vi "Main.vi"() -> ()   [LabVIEW 2017]
doc: "The myRIO Project template acquires acceleration data from the onboard accelerometer and displays the changes of acceleration values in a waveform chart."
uses:
  <vilib>/myRIO/Common/Instrument Driver Framework/myRIO v1.0/Encoder/typedefs/Encoder Count Direction Enum.ctl
  Motor Status Enum.ctl
  <vilib>/myRIO/Instrument Drivers/Onboard IO/PWM/typedefs/PWM Reference.ctl
  <vilib>/myRIO/Common/Instrument Driver Framework/Utilities/typedefs/myRIO Generic Hardware Reference.ctl
  <vilib>/myRIO/Common/Instrument Driver Framework/Utilities/typedefs/Hardware Version Enum.ctl
  <vilib>/myRIO/Common/Instrument Driver Framework/Utilities/typedefs/myRIO v1.0 Reference.ctl
  <vilib>/myRIO/Common/Instrument Driver Framework/Utilities/typedefs/Generic FPGA Reference.ctl
  <vilib>/myRIO/Common/Instrument Driver Framework/myRIO v1.0/PWM/typedefs/PWM Channels Enum.ctl
  <vilib>/myRIO/Instrument Drivers/Onboard IO/PWM/typedefs/PWM Configuration.ctl
  <vilib>/userdefined/High Color/nirio_resource_hc.ctl
  <vilib>/myRIO/Common/Instrument Driver Framework/Utilities/vis/Is FPGA Ref Available.vi
  <vilib>/myRIO/Common/Instrument Driver Framework/myRIO v1.0/PWM/vis/myRIO v1.1 Open PWM.vi
  <vilib>/myRIO/Instrument Drivers/Onboard IO/PWM/vis/Set Duty Cycle and Frequency.vi
  <vilib>/myRIO/Common/Instrument Driver Framework/Utilities/vis/Validate Channels.vi
  <vilib>/myRIO/Common/Instrument Driver Framework/myRIO v1.0/PWM/vis/myRIO v1.0 Reserve PWM.vi
  <vilib>/myRIO/Common/Instrument Driver Framework/myRIO v1.0/UART/vis/myRIO v1.0 Close UART.vi
  <vilib>/myRIO/Common/Instrument Driver Framework/myRIO v1.0/PWM/vis/myRIO v1.0 Build MUX Configuration PWM.vi
  <vilib>/myRIO/Common/Instrument Driver Framework/myRIO v1.0/Resource Manager/vis/myRIO v1.0 Reserve Channel List.vi
  <vilib>/myRIO/Common/Instrument Driver Framework/myRIO v1.0/Resource Manager/vis/myRIO v1.0 Create Configuration List.vi
  <vilib>/myRIO/Common/Instrument Driver Framework/myRIO v1.0/Resource Manager/vis/myRIO v1.0 Reserve Channel.vi
  <vilib>/myRIO/Common/Instrument Driver Framework/myRIO v1.0/Resource Manager/vis/myRIO v1.0 Unreserve Channel.vi
  <vilib>/myRIO/Common/Instrument Driver Framework/myRIO v1.0/Resource Manager/vis/myRIO v1.0 Build Mutex Name.vi
  <vilib>/Utility/VariantDataType/GetNumericInfo.vi
  <vilib>/Utility/error.llb/Error Cluster From Error Code.vi
  <vilib>/myRIO/Common/Instrument Driver Framework/myRIO v1.0/myRIO v1.1 Open.vi
  <vilib>/myRIO/Common/Instrument Driver Framework/Utilities/vis/IO Manager.vi
  <vilib>/myRIO/Common/Instrument Driver Framework/Utilities/vis/Configuration Manager.vi
  <vilib>/myRIO/Common/Instrument Driver Framework/myRIO v1.0/Resource Manager/vis/myRIO v1.0 Configure IO.vi
  <vilib>/myRIO/Common/Instrument Driver Framework/myRIO v1.0/myRIO v1.0 Close.vi
  <vilib>/myRIO/Common/Instrument Driver Framework/myRIO v1.0/PWM/vis/myRIO v1.0 Write PWM.vi
  <vilib>/myRIO/Common/Instrument Driver Framework/Utilities/vis/FPGA Ref Manager.vi
  <vilib>/myRIO/Common/Instrument Driver Framework/myRIO v1.0/myRIO v1.0 Reset FPGA.vi
  <vilib>/myRIO/Common/Instrument Driver Framework/myRIO v1.0/IRQ/vis/myRIO v1.0 IRQ Info FGV.vi
  <vilib>/myRIO/Common/Instrument Driver Framework/myRIO v1.0/IRQ/vis/myRIO v1.0 Timer IRQ Info FGV.vi
  <vilib>/myRIO/Common/Instrument Driver Framework/myRIO v1.0/IRQ/vis/myRIO v1.0 ISR Agent.vi
  <vilib>/myRIO/Express VI/Onboard IO/PWM/PWM Express VI.xnode
  <vilib>/myRIO/Instrument Drivers/Onboard IO/PWM/vis/myRIO PWM Open.xnode
  <vilib>/myRIO/Instrument Drivers/Utilities/Utilities.lvlib
  <vilib>/myRIO/Instrument Drivers/Onboard IO/PWM/PWM.lvlib
panel:
  out "X Axis state":T1
  out "Y Axis state":T1
  out "Loop Runtime (s)":dbl format="%.3f"
  in  "Clear Chart History":bool
  in  "Coordinates Input":cluster{"X-axis (mm)":dbl, "Y-axis (mm)":dbl}
  out "Y Axis":T2(graph)
  out "X Axis":T2(graph)
  in  "X Axis Motor Target":T3
  out "X Axis Motor Params":T4
  in  "Y Axis Motor Target":T5
  out "Y Axis Motor Params":T5
  in  "stop":bool
  out "Output String":string
  out "Encoder Output":T7
  out "Total Runtime (s)":dbl format="%.2f"
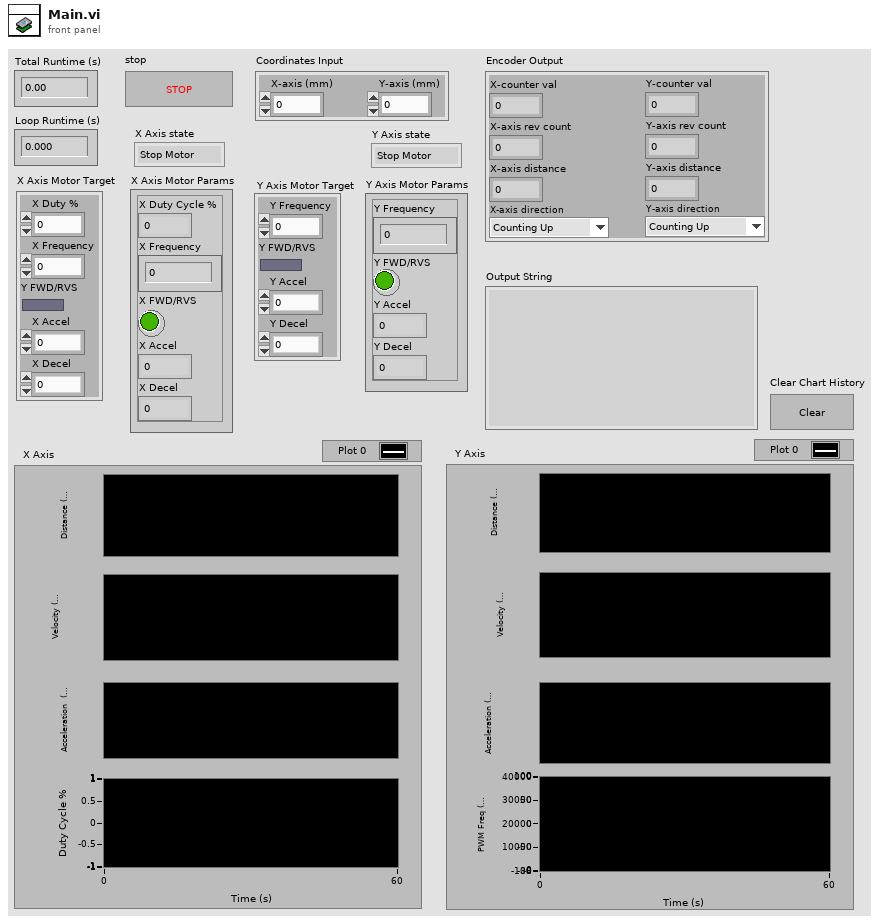
[diagram p1: front panel]
types:
  T1 = typedef "Motor Status Enum.ctl" = enum16{"Stop Motor", "Read Inputs", "Steady Speed", "Accelerate", "Decelerate"}
  T2 = cluster{"X-axis distance":dbl, dbl, dbl, "X Frequency":dbl}
  T3 = cluster{"X Frequency":dbl, "Y FWD/RVS":bool, "X Accel":dbl, "X Decel":dbl, "X Duty %":dbl}
  T4 = cluster{"X Frequency":dbl, "X FWD/RVS":bool, "X Accel":dbl, "X Decel":dbl, "X Duty Cycle %":dbl}
  T5 = cluster{"Y Frequency":dbl, "Y FWD/RVS":bool, "Y Accel":dbl, "Y Decel":dbl}
  T6 = typedef "Encoder Count Direction Enum.ctl" = enum16{"Counting Up", "Counting Down"}
  T7 = cluster{"Y-axis rev count":dbl, "Y-axis distance":dbl, "X-axis rev count":dbl, "X-axis distance":dbl, "Y-axis direction":T6, "X-axis direction":T6, "X-counter val":i32, "Y-counter val":i32}
  T8 = cluster{"X-axis distance":dbl, dbl, dbl, "X Frequency":dbl}[]
  T9 = cluster{dbl, dbl, "X-axis distance":dbl, "X Duty Cycle %":dbl, "X Frequency":dbl, "Y-axis distance":dbl, "Y Frequency":dbl, "X Accel":dbl, "X Decel":dbl, "Y Accel":dbl, "Y Decel":dbl, "X-axis (mm)":dbl, "Y-axis (mm)":dbl, dbl, dbl, dbl, dbl}
  T10 = cluster{"X-axis distance":dbl, dbl, dbl, "X Duty Cycle %":dbl}
  T11 = cluster{"Y-axis distance":dbl, dbl, dbl, "Y Frequency":dbl}
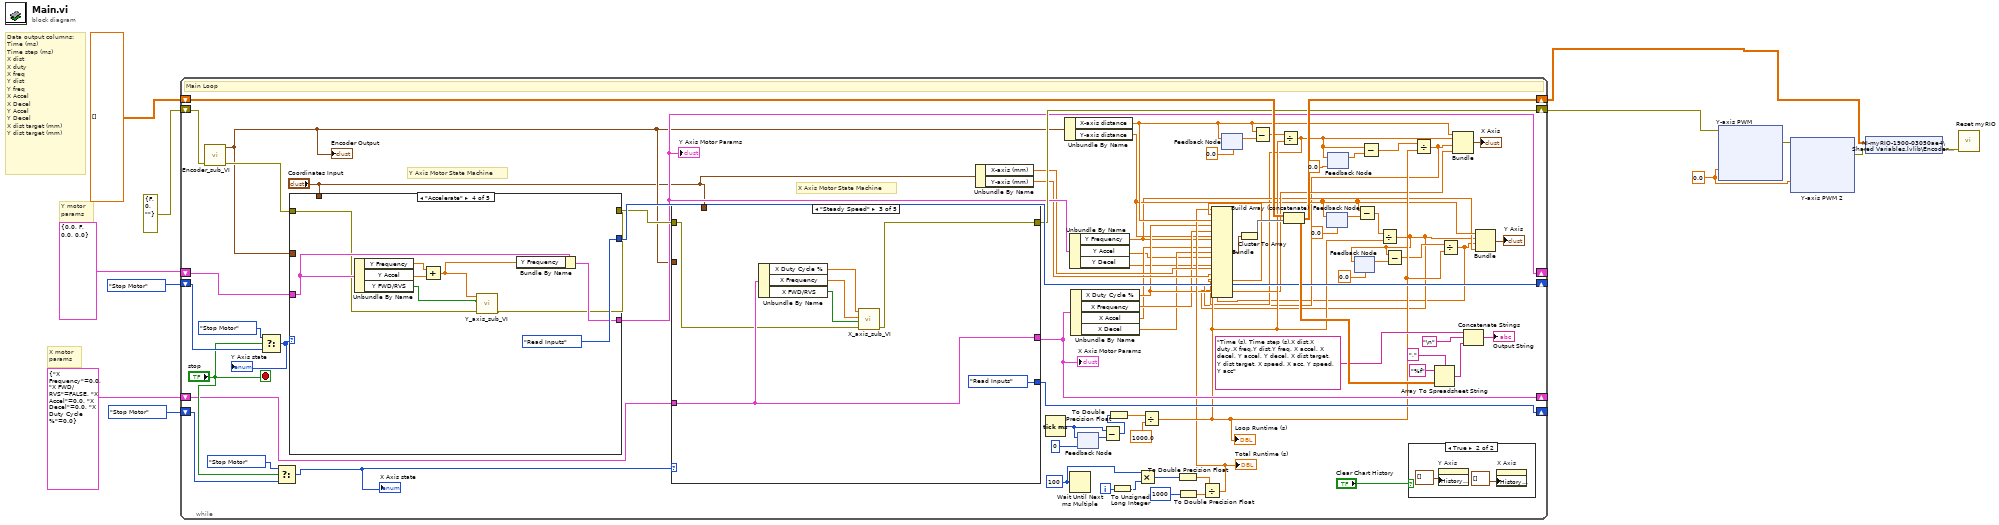
[diagram p0: block diagram]
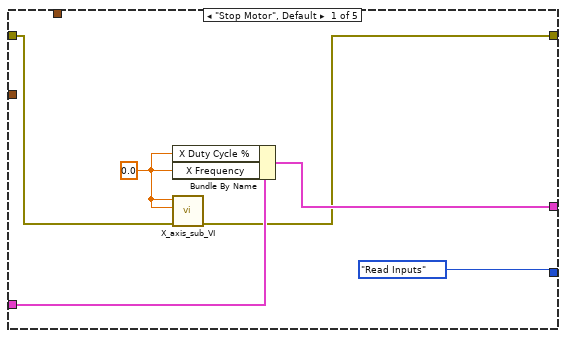
[diagram p3: hidden frame]
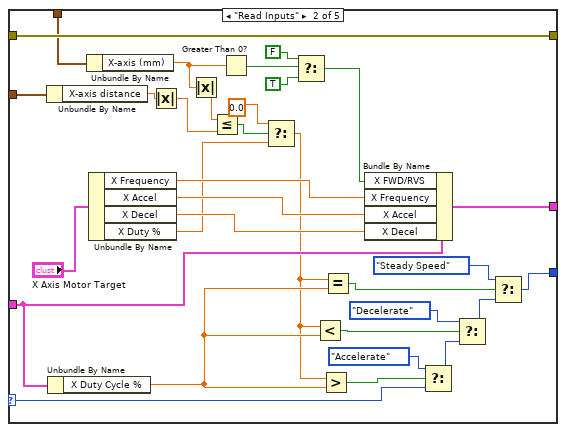
[diagram p4: hidden frame]
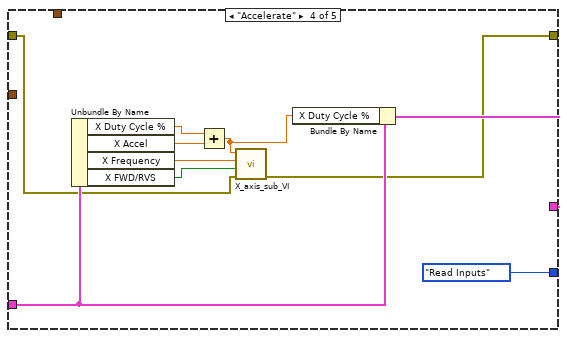
[diagram p5: hidden frame]
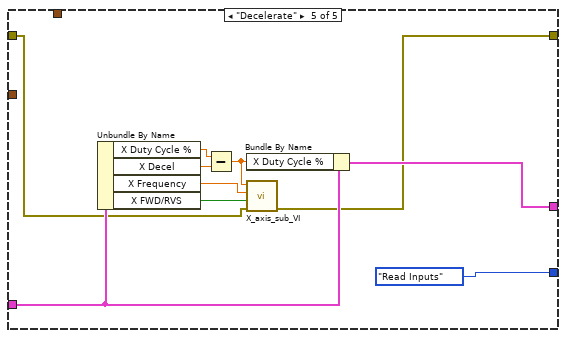
[diagram p6: hidden frame]
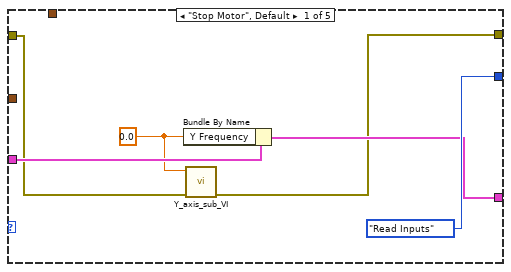
[diagram p7: hidden frame]
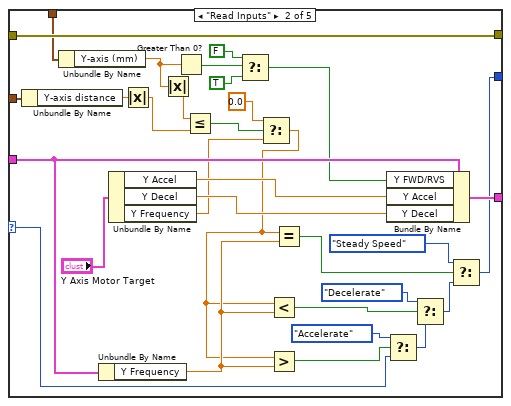
[diagram p8: hidden frame]
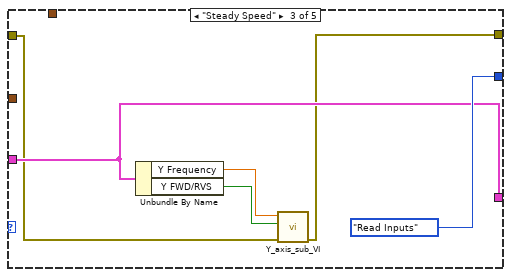
[diagram p9: hidden frame]
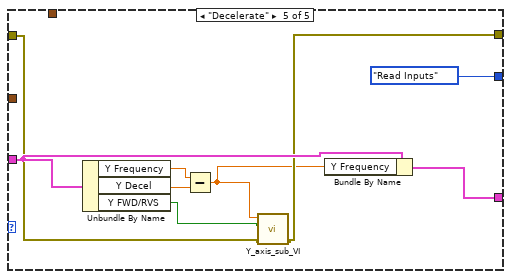
[diagram p10: hidden frame]
diagram:
  w6 = 0.0 ("Frequency [Hz]")
  # "X motor \nparams"
  # "Y motor \nparams"
  # "Data output columns:\nTime (ms)\nTime step (ms)\nX dist\nX duty\nX freq\nY dist\nY freq\nX Accel\nX Decel\nY Accel\nY Decel\nX dist target (mm)\nY dist target (mm)"
  n1 = while {
    shift-right: [w68] -> w12
    shift-left: errorcluster {"status"=FALSE, "code"=0, "source"=""} ("error in (no error)") -> [w86]
    shift-right: [w83] -> w1
    shift-left: dbl[][] [] -> [w82]
    shift-right: [w60] -> _
    shift-left: T5 {"Y Frequency"=0.0, "Y FWD/RVS"=FALSE, "Y Accel"=0.0, "Y Decel"=0.0} ("Y Axis Motor Params 2") -> [w81]
    shift-right: [w80] -> _
    shift-left: Motor_Status_Enum."Stop Motor" -> [w78]
    shift-right: [w71] -> _
    shift-left: Motor_Status_Enum."Stop Motor" -> [w73]
    shift-right: [w61] -> _
    shift-left: T4 {"X Frequency"=0.0, "X FWD/RVS"=FALSE, "X Accel"=0.0, "X Decel"=0.0, "X Duty Cycle %"=0.0} ("X Axis Motor Params 3") -> [w70]
    i -> [w32]
    stop <- "stop" stop-if-true
    w31 = u32 100 ("milliseconds to wait")
    # "X Axis Motor State Machine"
    # "Y Axis Motor State Machine"
    # "Main Loop"
    n2 = call "Encoder_sub_VI.vi"("error in (no error)"=w86) -> ("error out"=w76:errorcluster, "Encoder Output"=w59:T7)  [unwired: 9 in]
    "Encoder Output" <- w59
    n3 = Select(t=Motor_Status_Enum."Stop Motor", s="stop", f=w78) -> (s? t:f=w79:T1)
    "Y Axis state" <- w79
    n4 = Select(t=Motor_Status_Enum."Stop Motor", s="stop", f=w73) -> (s? t:f=w74:T1)
    "X Axis state" <- w74
    n5 = case shown="\"Accelerate\"" w79 {
      selector: w79 -> [_ w176 _ _ _]
      tunnel: w81 -> [w159 w177 w193 w202 w210]
      tunnel: [Motor_Status_Enum."Read Inputs" w160 Motor_Status_Enum."Read Inputs" Motor_Status_Enum."Read Inputs" Motor_Status_Enum."Read Inputs"] -> w80
      tunnel: [w157 w178 w193 w201 w211] -> w60
      tunnel: w76 -> [w155 w175 w192 w198 w208]
      tunnel: [w156 w175 w191 w197 w209] -> w69
      tunnel: w59 -> [_ w174 _ _ _]
      tunnel: "Coordinates Input" -> [_ w170 _ _ _]
      frame "Stop Motor", Default {
        w154 = 0.0 ("Y Frequency")
        n6 = Bundle By Name(cluster=w159, "Y Frequency"=w154) -> (w157:T5)
        n7 = call "Y_axis_sub_VI.vi"("error in (no error)"=w155, "Frequency"=w154) -> ("error out"=w156:errorcluster)  [unwired: 9 in]
      }
      frame "Read Inputs" {
        n8 = Unbundle By Name(w174) -> ("Y-axis distance"=w168:dbl)
        n9 = Unbundle By Name(w170) -> ("Y-axis (mm)"=w167:dbl)
        n10 = Unbundle By Name(w177) -> ("Y Frequency"=w184:dbl)
        n11 = Unbundle By Name("Y Axis Motor Target") -> ("Y Accel"=w188:dbl, "Y Decel"=w189:dbl, "Y Frequency"=w162:dbl)
        n12 = Absolute Value(x=w168) -> (abs(x)=w165:dbl)
        n13 = Absolute Value(x=w167) -> (abs(x)=w166:dbl)
        n14 = Greater Than 0?(x=w167) -> (x > 0?=w169:bool)
        n15 = Less Or Equal?(x=w166, y=w165) -> (x <= y?=w164:bool)
        n16 = Select(t=FALSE, s=w169, f=TRUE) -> (s? t:f=w171:bool)
        n17 = Select(t=0.0, s=w164, f=w162) -> (s? t:f=w161:dbl)
        n18 = Less?(x=w161, y=w184) -> (x < y?=w181:bool)
        n19 = Greater?(x=w161, y=w184) -> (0:w190:bool)
        n20 = Equal?(x=w161, y=w184) -> (x = y?=w185:bool)
        n21 = Bundle By Name(cluster=w177, "Y FWD/RVS"=w171, "Y Accel"=w188, "Y Decel"=w189) -> (w178:T5)
        n22 = Select(t=Motor_Status_Enum."Accelerate", s=w190, f=w176) -> (s? t:f=w183:T1)
        n23 = Select(t=Motor_Status_Enum."Decelerate", s=w181, f=w183) -> (s? t:f=w186:T1)
        n24 = Select(t=Motor_Status_Enum."Steady Speed", s=w185, f=w186) -> (s? t:f=w160:T1)
      }
      frame "Steady Speed" {
        n25 = Unbundle By Name(w193) -> ("Y Frequency"=w195:dbl, "Y FWD/RVS"=w196:bool)
        n26 = call "Y_axis_sub_VI.vi"("error in (no error)"=w192, "FWD/RVS"=w196, "Frequency"=w195) -> ("error out"=w191:errorcluster)  [unwired: 8 in]
      }
      frame "Accelerate" {
        n27 = Unbundle By Name(w202) -> ("Y Frequency"=w204:dbl, "Y Accel"=w205:dbl, "Y FWD/RVS"=w199:bool)
        n28 = Add(x=w204, y=w205) -> (x+y=w200:dbl)
        n29 = call "Y_axis_sub_VI.vi"("error in (no error)"=w198, "FWD/RVS"=w199, "Frequency"=w200) -> ("error out"=w197:errorcluster)  [unwired: 8 in]
        n30 = Bundle By Name(cluster=w202, "Y Frequency"=w200) -> (w201:T5)
      }
      frame "Decelerate" {
        n31 = Unbundle By Name(w210) -> ("Y Frequency"=w214:dbl, "Y Decel"=w213:dbl, "Y FWD/RVS"=w207:bool)
        n32 = Subtract(x=w214, y=w213) -> (x-y=w206:dbl)
        n33 = call "Y_axis_sub_VI.vi"("error in (no error)"=w208, "FWD/RVS"=w207, "Frequency"=w206) -> ("error out"=w209:errorcluster)  [unwired: 8 in]
        n34 = Bundle By Name(cluster=w210, "Y Frequency"=w206) -> (w211:T5)
      }
    }
    "Y Axis Motor Params" <- w60
    n35 = case shown="\"Steady Speed\"" w74 {
      selector: w74 -> [_ w114 _ _ _]
      tunnel: [Motor_Status_Enum."Read Inputs" w107 Motor_Status_Enum."Read Inputs" Motor_Status_Enum."Read Inputs" Motor_Status_Enum."Read Inputs"] -> w71
      tunnel: [w91 w113 w130 w137 w147] -> w61
      tunnel: w70 -> [w92 w112 w130 w136 w146]
      tunnel: w69 -> [w90 w110 w128 w135 w145]
      tunnel: [w89 w110 w127 w134 w144] -> w68
      tunnel: w59 -> [_ w109 _ _ _]
      tunnel: "Coordinates Input" -> [_ w108 _ _ _]
      frame "Stop Motor", Default {
        w94 = 0.0 ("Y Frequency")
        n36 = Bundle By Name(cluster=w92, "X Duty Cycle %"=w94, "X Frequency"=w94) -> (w91:T4)
        n37 = call "X_axis_sub_VI.vi"("error in (no error)"=w90, "Frequency"=w94, "Duty Cycle %"=w94) -> ("error out"=w89:errorcluster)  [unwired: 8 in]
      }
      frame "Read Inputs" {
        n38 = Unbundle By Name(w109) -> ("X-axis distance"=w101:dbl)
        n39 = Unbundle By Name(w112) -> ("X Duty Cycle %"=w125:dbl)
        n40 = Unbundle By Name(w108) -> ("X-axis (mm)"=w99:dbl)
        n41 = Unbundle By Name("X Axis Motor Target") -> ("X Frequency"=w117:dbl, "X Accel"=w115:dbl, "X Decel"=w116:dbl, "X Duty %"=w97:dbl)
        n42 = Absolute Value(x=w101) -> (abs(x)=w100:dbl)
        n43 = Absolute Value(x=w99) -> (abs(x)=w104:dbl)
        n44 = Less Or Equal?(x=w104, y=w100) -> (x <= y?=w103:bool)
        n45 = Greater Than 0?(x=w99) -> (x > 0?=w105:bool)
        n46 = Select(t=0.0, s=w103, f=w97) -> (s? t:f=w96:dbl)
        n47 = Select(t=FALSE, s=w105, f=TRUE) -> (s? t:f=w98:bool)
        n48 = Less?(x=w96, y=w125) -> (x < y?=w120:bool)
        n49 = Greater?(x=w96, y=w125) -> (0:w118:bool)
        n50 = Equal?(x=w96, y=w125) -> (x = y?=w124:bool)
        n51 = Bundle By Name(cluster=w112, "X FWD/RVS"=w98, "X Frequency"=w117, "X Accel"=w115, "X Decel"=w116) -> (w113:T4)
        n52 = Select(t=Motor_Status_Enum."Accelerate", s=w118, f=w114) -> (s? t:f=w122:T1)
        n53 = Select(t=Motor_Status_Enum."Decelerate", s=w120, f=w122) -> (s? t:f=w123:T1)
        n54 = Select(t=Motor_Status_Enum."Steady Speed", s=w124, f=w123) -> (s? t:f=w107:T1)
      }
      frame "Steady Speed" {
        n55 = Unbundle By Name(w130) -> ("X Duty Cycle %"=w132:dbl, "X Frequency"=w131:dbl, "X FWD/RVS"=w133:bool)
        n56 = call "X_axis_sub_VI.vi"("error in (no error)"=w128, "FWD/RVS"=w133, "Frequency"=w131, "Duty Cycle %"=w132) -> ("error out"=w127:errorcluster)  [unwired: 7 in]
      }
      frame "Accelerate" {
        n57 = Unbundle By Name(w136) -> ("X Duty Cycle %"=w139:dbl, "X Accel"=w140:dbl, "X Frequency"=w141:dbl, "X FWD/RVS"=w143:bool)
        n58 = Add(x=w139, y=w140) -> (x+y=w142:dbl)
        n59 = call "X_axis_sub_VI.vi"("error in (no error)"=w135, "FWD/RVS"=w143, "Frequency"=w141, "Duty Cycle %"=w142) -> ("error out"=w134:errorcluster)  [unwired: 7 in]
        n60 = Bundle By Name(cluster=w136, "X Duty Cycle %"=w142) -> (w137:T4)
      }
      frame "Decelerate" {
        n61 = Unbundle By Name(w146) -> ("X Duty Cycle %"=w149:dbl, "X Decel"=w150:dbl, "X Frequency"=w151:dbl, "X FWD/RVS"=w153:bool)
        n62 = Subtract(x=w149, y=w150) -> (x-y=w152:dbl)
        n63 = Bundle By Name(cluster=w146, "X Duty Cycle %"=w152) -> (w147:T4)
        n64 = call "X_axis_sub_VI.vi"("error in (no error)"=w145, "FWD/RVS"=w153, "Frequency"=w151, "Duty Cycle %"=w152) -> ("error out"=w144:errorcluster)  [unwired: 7 in]
      }
    }
    "X Axis Motor Params" <- w61
    n65 = Unbundle By Name("Coordinates Input") -> ("X-axis (mm)"=w25:dbl, "Y-axis (mm)"=w50:dbl)
    n66 = Tick Count (ms)() -> (millisecond timer value=w49:u32)
    n67 = Unbundle By Name(w59) -> ("X-axis distance"=w46:dbl, "Y-axis distance"=w20:dbl)
    n68 = Unbundle By Name(w60) -> ("Y Frequency"=w19:dbl, "Y Accel"=w18:dbl, "Y Decel"=w17:dbl)
    n69 = Wait Until Next ms Multiple(millisecond multiple=w31) -> ()  [unwired: 1 out]
    n70 = Unbundle By Name(w61) -> ("X Duty Cycle %"=w24:dbl, "X Frequency"=w23:dbl, "X Accel"=w22:dbl, "X Decel"=w21:dbl)
    n71 = feedback-in #1(w49) -> ()
    n72 = feedback #1(u32 0) -> (w48:u32)
    n73 = Subtract(x=w49, y=w48) -> (x-y=w54:u32)
    n74 = To Double Precision Float(number=w54) -> (double precision float=w52:dbl)
    n75 = To Unsigned Long Integer(number=w32) -> (unsigned 32bit integer=w30:u32)
    n76 = Multiply(x=w31, y=w30) -> (x*y=w29:u32)
    n77 = Divide(x=w52, y=1000.0) -> (x/y=w37:dbl)
    "Loop Runtime (s)" <- w37
    n78 = To Double Precision Float(number=w29) -> (double precision float=w27:dbl)
    n79 = To Double Precision Float(number=u32 1000 ("y")) -> (double precision float=w26:dbl)
    n80 = Divide(x=w27, y=w26) -> (x/y=w28:dbl)
    "Total Runtime (s)" <- w28
    n81 = feedback #2(0.0) -> (w45:dbl)
    n82 = feedback-in #2(w46) -> ()
    n83 = Subtract(x=w46, y=w45) -> (x-y=w44:dbl)
    n84 = Divide(x=w44, y=w37) -> (x/y=w16:dbl)
    n85 = feedback #3(0.0) -> (w40:dbl)
    n86 = feedback-in #3(w20) -> ()
    n87 = feedback #4(0.0) -> (w43:dbl)
    n88 = feedback-in #4(w16) -> ()
    n89 = feedback #5(0.0) -> (w35:dbl)
    n90 = Subtract(x=w20, y=w40) -> (x-y=w38:dbl)
    n91 = Subtract(x=w16, y=w43) -> (x-y=w41:dbl)
    n92 = Divide(x=w38, y=w37) -> (x/y=w14:dbl)
    n93 = feedback-in #5(w14) -> ()
    n94 = Subtract(x=w14, y=w35) -> (x-y=w34:dbl)
    n95 = case shown="True" "Clear Chart History" {
      frame False {
      }
      frame True {
        n96 = property on="Y Axis" class="WFChart (strict)"("History Data"=T8 []) -> ()  [unwired: 2 in, 2 out]
        n97 = property on="X Axis" class="WFChart (strict)"("History Data"=T8 []) -> ()  [unwired: 2 in, 2 out]
      }
    }
    n98 = Divide(x=w41, y=w37) -> (x/y=w15:dbl)
    n99 = Divide(x=w34, y=w37) -> (x/y=w13:dbl)
    n100 = Bundle(w28, w37, "X-axis distance"=w46, "X Duty Cycle %"=w24, "X Frequency"=w23, "Y-axis distance"=w20, "Y Frequency"=w19, "X Accel"=w22, "X Decel"=w21, "Y Accel"=w18, "Y Decel"=w17, "X-axis (mm)"=w25, "Y-axis (mm)"=w50, w16, w15, w14, w13) -> (w84:T9)  [unwired: 1 in]
    n101 = Cluster To Array(cluster=w84) -> (array=w85:dbl[])
    n102 = Build Array (concatenate)(w82, w85) -> (w83:dbl[][])
    n103 = Array To Spreadsheet String(delimiter (Tab)=",", array=w83, 3:"%f" ("format string")) -> (spreadsheet string=w66:string)
    n104 = Bundle("X-axis distance"=w46, w16, w15, "X Duty Cycle %"=w24) -> (→"X Axis":T10)  [unwired: 1 in]
    n105 = Concatenate Strings("Time (s), Time step (s),X dist,X duty,X freq,Y dist,Y freq, X accel, X decel, Y accel, Y decel, X dist target, Y dist target, X speed, X acc, Y speed, Y acc", "\n", w66) -> (→"Output String":string)
    n106 = Bundle("Y-axis distance"=w20, w14, w13, "Y Frequency"=w19) -> (→"Y Axis":T11)  [unwired: 1 in]
  }
  n107 = xnode "Y-axis PWM"("Frequency [Hz]"=w6, "error in (no error)"=w12) -> ("error out"=w8:errorcluster)
  n108 = xnode "Y-axis PWM 2"("Frequency [Hz]"=w6, "error in (no error)"=w8) -> ("error out"=w7:errorcluster)
  n109 = shared-variable "NI-myRIO-1900-03050ae4\\Shared Variables.lvlib\\Encoder Data"(w1, error in=w7) -> (error out=w9:errorcluster)
  n110 = call <vilib>:"Reset myRIO.vi"("error in (no error)"=w9) -> ()  [unwired: 10 in, 1 out]
